vi "clear.vi"(8 "error in (no error)":errorcluster) -> (0 "error out":errorcluster)   [LabVIEW 2024, in "controls manager.lvlib"]
uses:
  controls manager.lvlib
  fgv actions.ctl
  <vilib>/Utility/error.llb/Error Cluster From Error Code.vi
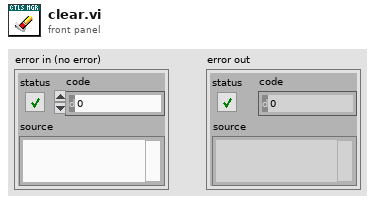
[diagram p1: front panel]
types:
  T1 = typedef "controls manager.lvlib/fgv actions.ctl" = enum16{"create", "get", "destroy"}
  T2 = typedef "controls manager.lvlib/collection type.ctl" = map{string, T3}
  T3 = typedef "controls manager.lvlib/entry type.ctl" = cluster{"controls":map{string, T4}, "plan":T5}
  T4 = typedef "controls manager.lvlib/control.ctl" = cluster{"refnum":refnum<vi>, "index":i32}
  T5 = typedef "controls manager.lvlib/controls plan.ctl" = map{string, T6[]}
  T6 = typedef "controls manager.lvlib/key value pair.ctl" = cluster{"key":string, "value":string}
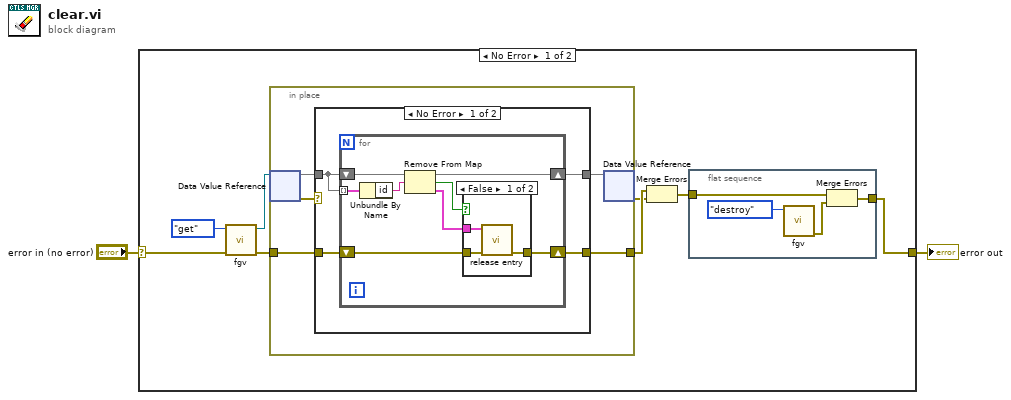
[diagram p0: block diagram]
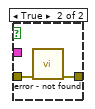
[diagram p2: hidden frame]
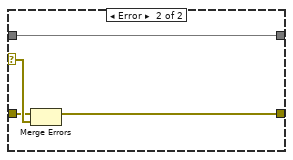
[diagram p3: hidden frame]
diagram:
  n1 = case shown="No Error" "error in (no error)" {
    selector: "error in (no error)" -> [w5 w41]
    tunnel: [w7 w41] -> w1
    frame No Error {
      n2 = call "fgv.vi"("error in (no error)"=w5, "action"=fgv_actions."get") -> ("error out"=w4:errorcluster, "dvr"=w6:refnum<data-value>)  [unwired: 8 in]
      n3 = in-place {
        in-place-border: w4 -> [w17]
        in-place-border: [w16] -> w10
        n4 = in-place-dvr #1(w6) -> (w19:T2, w15:errorcluster)
        n5 = case shown="No Error" w15 {
          selector: w15 -> [_ w39]
          tunnel: w19 -> [w20 w40]
          tunnel: [w23 w40] -> w18
          tunnel: w17 -> [w22 w38]
          tunnel: [w21 w37] -> w16
          frame No Error {
            n6 = for {
              shift-right: [w28] -> w21
              shift-left: w22 -> [w29]
              tunnel: w20 -> [w25] mode=indexing
              shift-right: [w30] -> w23
              shift-left: w20 -> [w31]
              n7 = Unbundle By Name(w25) -> ("id"=w24:string)
              n8 = Remove From Map(10:w24, 11:w31) -> (1:w27:T3, 2:w26:bool, 3:w30:T2)
              n9 = case shown="False" w26 {
                tunnel: w27 -> [w34 _]
                tunnel: w29 -> [w33 w36]
                tunnel: [w32 w35] -> w28
                frame False {
                  n10 = call "release entry.vi"("error in (no error)"=w33, "entry"=w34) -> ("error out"=w32:errorcluster)  [unwired: 9 in]
                }
                frame True {
                  n11 = call "error - not found.vi"("error in (no error)"=w36) -> ("error out"=w35:errorcluster)  [unwired: 10 in]
                }
              }
            }
          }
          frame Error {
            n12 = Merge Errors(w38, w39) -> (w37:errorcluster)
          }
        }
        n13 = in-place-dvr #1(w18) -> (w9:errorcluster)  [unwired: 1 out]
      }
      n14 = Merge Errors(w10, w9) -> (w8:errorcluster)
      n15 = flat-sequence {
        tunnel: w8 -> [w14]
        tunnel: [w13] -> w7
        frame #0 {
          n16 = call "fgv.vi"("action"=fgv_actions."destroy") -> ("error out"=w11:errorcluster)  [unwired: 9 in, 1 out]
          n17 = Merge Errors(w14, w11) -> (w13:errorcluster)
        }
      }
    }
    frame Error {
    }
  }
  "error out" <- w1
